vi "CALCULATE_ISP.vi"(5 "Thrust":waveform(dbl), 7 "Oxidizer Temperature":waveform(dbl), 8 "Oxidizer Type":enum16{"LOX", "Water", "Nitrogen"}(ring), 9 "Fuel Type":enum16{"RP1", "Biodiesel", "Water"}(ring), 10 "Oxidizer Flow Rate":dbl, 11 "Fuel Flow Rate":dbl) -> (3 "Specific Impulse":waveform(dbl))   [LabVIEW 2013]
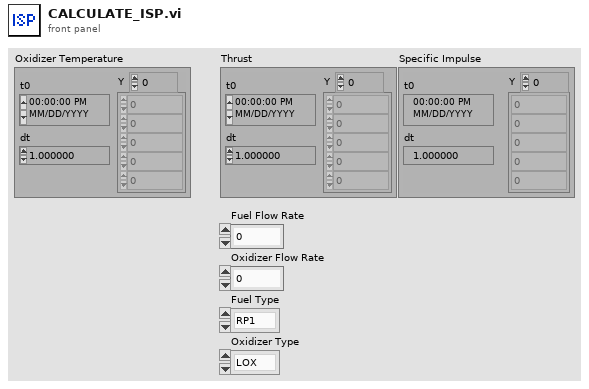
[diagram p1: front panel]
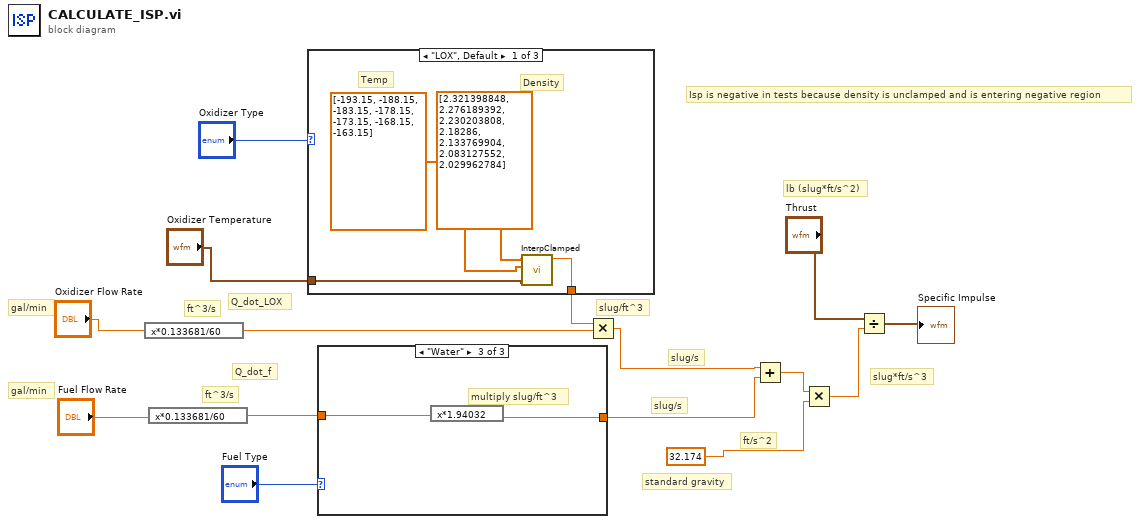
[diagram p0: block diagram]
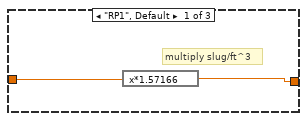
[diagram p2: hidden frame]
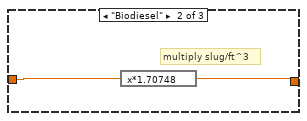
[diagram p3: hidden frame]
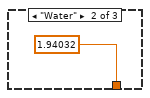
[diagram p4: hidden frame]
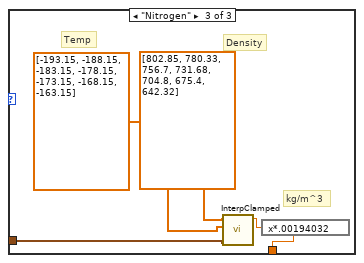
[diagram p5: hidden frame]
diagram:
  # "Isp is negative in tests because density is unclamped and is entering negative region"
  # "slug*ft/s^3"
  # "ft/s^2"
  # "slug/s"
  # "slug/s"
  # "slug/ft^3"
  # "Q_dot_LOX"
  # "Q_dot_f"
  # "ft^3/s"
  # "ft^3/s"
  # "lb (slug*ft/s^2)"
  # "gal/min"
  # "gal/min"
  # "standard gravity"
  n1 = expression code="x*0.133681/60"("Oxidizer Flow Rate") -> (w4:dbl)
  n2 = expression code="x*0.133681/60"("Fuel Flow Rate") -> (w8:dbl)
  n3 = case shown="\"LOX\", Default" "Oxidizer Type" {
    tunnel: [w16 1.94032 w25] -> w5
    tunnel: "Oxidizer Temperature" -> [w17 _ w23]
    frame "LOX", Default {
      # "Density"
      # "Temp"
      n4 = call "InterpClamped.vi"("x value"=w17, "X"=dbl[] [-193.15, -188.15, -183.15, -178.15, -173.15, -168.15, -163.15], "Y"=dbl[] [2.321398848, 2.276189392, 2.230203808, 2.18286, 2.133769904, 2.083127552, 2.029962784] ("X")) -> ("clamped value"=w16:dbl)  [unwired: 7 in, 1 out]
    }
    frame "Water" {
    }
    frame "Nitrogen" {
      # "kg/m^3"
      # "Density"
      # "Temp"
      n5 = call "InterpClamped.vi"("x value"=w23, "X"=dbl[] [-193.15, -188.15, -183.15, -178.15, -173.15, -168.15, -163.15], "Y"=dbl[] [802.85, 780.33, 756.7, 731.68, 704.8, 675.4, 642.32] ("X")) -> ("clamped value"=w24:dbl)  [unwired: 7 in, 1 out]
      n6 = expression code="x*.00194032"(w24) -> (w25:dbl)
    }
  }
  n7 = case shown="\"Water\"" "Fuel Type" {
    tunnel: w8 -> [w27 w28 w31]
    tunnel: [w26 w29 w30] -> w7
    frame "RP1", Default {
      # "multiply slug/ft^3"
      n8 = expression code="x*1.57166"(w27) -> (w26:dbl)
    }
    frame "Biodiesel" {
      # "multiply slug/ft^3"
      n9 = expression code="x*1.70748"(w28) -> (w29:dbl)
    }
    frame "Water" {
      # "multiply slug/ft^3"
      n10 = expression code="x*1.94032"(w31) -> (w30:dbl)
    }
  }
  n11 = Multiply(x=w5, y=w4) -> (x*y=w3:dbl)
  n12 = Add(x=w3, y=w7) -> (x+y=w14:dbl)
  n13 = Multiply(x=w14, y=32.174) -> (x*y=w13:dbl)
  n14 = Divide(x="Thrust", y=w13) -> (x/y=→"Specific Impulse":waveform(dbl))
